vi "VI Tree.vi"   [LabVIEW 2019, in "Tektronix AFG 3000 Series.lvlib"]
doc: "This is the instrument driver for the <B>Tektronix AFG 300 Series</B>. The VI Tree displays all the user-callable VIs of the instrument driver in an organized table."
uses:
  Tektronix AFG 3000 Series.lvlib
  Configure/Configure Modulation (Amplitude).vi
panel:
  # "(c) 2006-2019 National Instruments.  ALL RIGHTS RESERVED."
  # "SEE DIAGRAM\nFOR VI TREE."
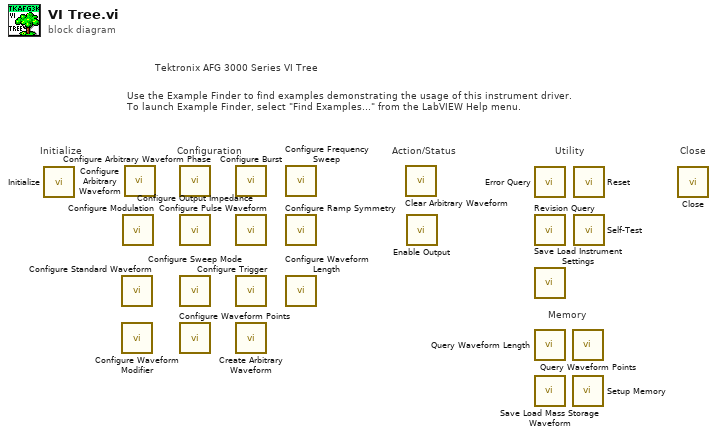
[diagram p0: block diagram]
diagram:
  # "Memory"
  # "Tektronix AFG 3000 Series VI Tree"
  # "Use the Example Finder to find examples demonstrating the usage of this instrument driver.\nTo launch Example Finder, select \"Find Examples...\" from the LabVIEW Help menu."
  # "Configuration"
  # "Utility"
  # "Action/Status"
  # "Close"
  # "Initialize"
  n1 = call "Initialize.vi"() -> ()  [unwired: 10 in, 2 out]
  n2 = call "Configure Standard Waveform.vi"() -> ()  [unwired: 14 in, 2 out]
  n3 = call "Configure Waveform Modifier.vi"() -> ()  [unwired: 10 in, 2 out]
  n4 = call-poly "Configure Modulation.vi"() -> ()  [unwired: 14 in, 2 out]
  n5 = call "Configure Arbitrary Waveform.vi"() -> ()  [unwired: 10 in, 2 out]
  n6 = call "Configure Arbitrary Waveform Phase.vi"() -> ()  [unwired: 10 in, 2 out]
  n7 = call "Configure Output Impedance.vi"() -> ()  [unwired: 10 in, 2 out]
  n8 = call "Configure Sweep Mode.vi"() -> ()  [unwired: 10 in, 2 out]
  n9 = call "Configure Waveform Points.vi"() -> ()  [unwired: 10 in, 2 out]
  n10 = call "Configure Burst.vi"() -> ()  [unwired: 10 in, 2 out]
  n11 = call "Configure Pulse Waveform.vi"() -> ()  [unwired: 10 in, 2 out]
  n12 = call "Configure Trigger.vi"() -> ()  [unwired: 10 in, 2 out]
  n13 = call "Create Arbitrary Waveform.vi"() -> ()  [unwired: 10 in, 2 out]
  n14 = call "Configure Frequency Sweep.vi"() -> ()  [unwired: 14 in, 2 out]
  n15 = call "Configure Ramp Symmetry.vi"() -> ()  [unwired: 10 in, 2 out]
  n16 = call "Configure Waveform Length.vi"() -> ()  [unwired: 10 in, 2 out]
  n17 = call "Clear Arbitrary Waveform.vi"() -> ()  [unwired: 10 in, 2 out]
  n18 = call "Enable Output.vi"() -> ()  [unwired: 10 in, 2 out]
  n19 = call "Error Query.vi"() -> ()  [unwired: 8 in, 4 out]
  n20 = call "Revision Query.vi"() -> ()  [unwired: 8 in, 4 out]
  n21 = call "Save Load Instrument Settings.vi"() -> ()  [unwired: 10 in, 2 out]
  n22 = call "Query Waveform Length.vi"() -> ()  [unwired: 9 in, 3 out]
  n23 = call "Save Load Mass Storage Waveform.vi"() -> ()  [unwired: 10 in, 2 out]
  n24 = call "Query Waveform Points.vi"() -> ()  [unwired: 9 in, 3 out]
  n25 = call "Setup Memory.vi"() -> ()  [unwired: 9 in, 3 out]
  n26 = call "Reset.vi"() -> ()  [unwired: 10 in, 2 out]
  n27 = call "Self-Test.vi"() -> ()  [unwired: 8 in, 4 out]
  n28 = call "Close.vi"() -> ()  [unwired: 11 in, 1 out]
